vi "Device Pre Install Tasks.vi"(8 "Error In":errorcluster, 11 "Install LV Data":T1) -> (0 "Error Out":errorcluster, 3 "Install LV Data":T1={"SSH Session"=refnum, "Status Log"="", "Detailed Log"="", "Credentials"={"Hostname or IP"="192.168.7.2", "Username"="root", "Password"=""}, "Target Info"={"OS Version"="", "CPU"="", "Systemd Version"="", "Internet Access"=FALSE, "Device Type"="", "LV Installed Ver"="", "LV Available Ver"="", "LV Upgrade Available"=FALSE, "Hostname"="", "NIC Info"=[]}, "Reboot Required?"=FALSE})   [LabVIEW 2014, in "LMH-LINX.lvlib"]
uses:
  <vilib>/MakerHub/LINX/LMH-LINX.lvlib
  <vilib>/MakerHub/LINX/Private/Utilties/Target Management/Install LV Data.ctl
  C:/Program Files (x86)/National Instruments/LabVIEW 2014/vi.lib/MakerHub/LINX/Resources/Renci.SshNet.dll
  Resources/Renci.SshNet.dll
  <vilib>/MakerHub/LINX/Private/Utilties/Target Management/Target Info.ctl
  <vilib>/MakerHub/LINX/Private/Utilties/Target Management/NIC Info.ctl
  <vilib>/MakerHub/LINX/Private/Utilties/Target Management/NIC Mode.ctl
  <vilib>/MakerHub/LINX/Private/Utilties/Target Management/Status FGV States.ctl
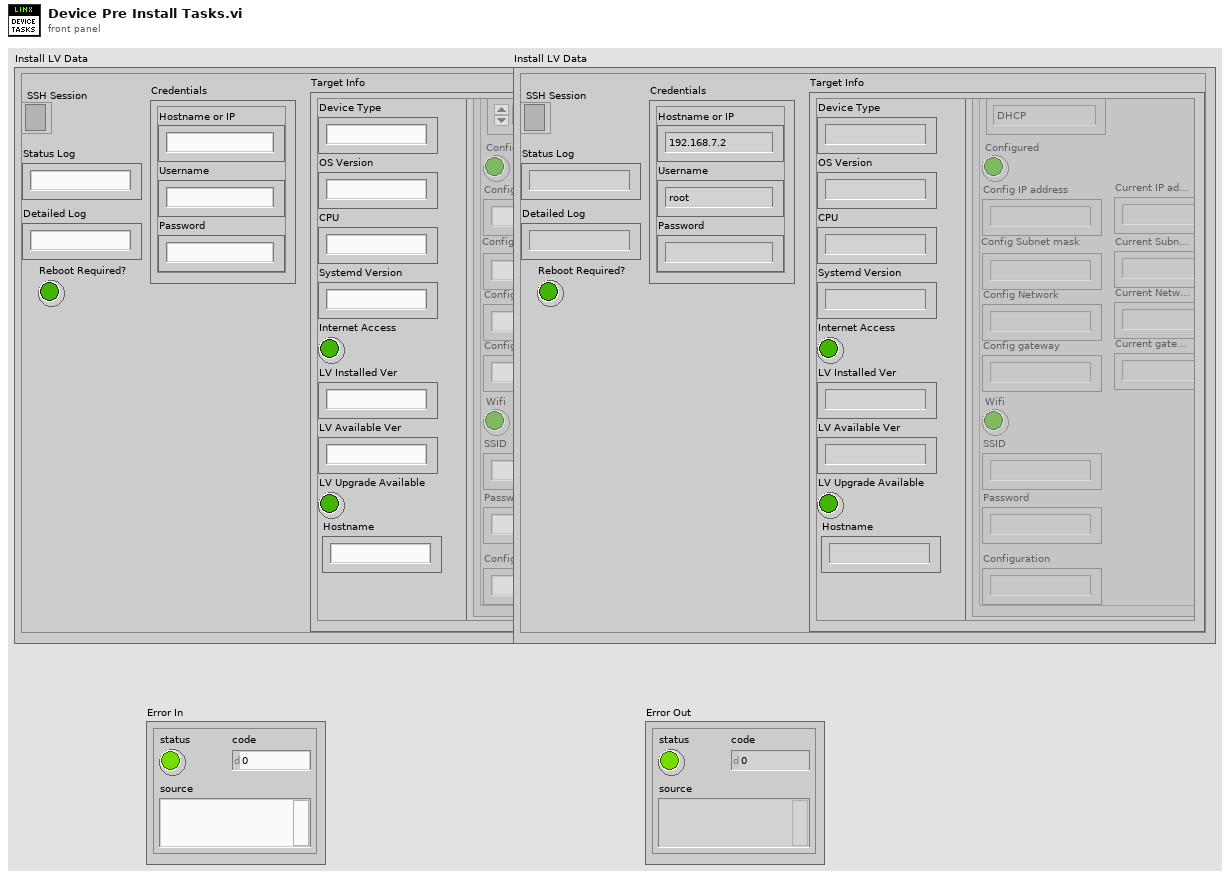
[diagram p1: front panel]
types:
  T1 = typedef "LMH-LINX.lvlib/Install LV Data.ctl" = cluster{"SSH Session":refnum<k24>, "Status Log":string, "Detailed Log":string, "Credentials":cluster{"Hostname or IP":string, "Username":string, "Password":string}, "Target Info":T2, "Reboot Required?":bool}
  T2 = typedef "LMH-LINX.lvlib/Target Info.ctl" = cluster{"OS Version":string, "CPU":string, "Systemd Version":string, "Internet Access":bool, "Device Type":string, "LV Installed Ver":string, "LV Available Ver":string, "LV Upgrade Available":bool, "Hostname":string, "NIC Info":T3[]}
  T3 = typedef "LMH-LINX.lvlib/NIC Info.ctl" = cluster{"Name":string, "NIC Mode":T4, "Configured":bool, "Config IP address":string, "Config Subnet mask":string, "Config Network":string, "Config gateway":string, "Wifi":bool, "SSID":string, "Password":string, "Configuration":string, "Current IP address":string, "Current Subnet mask":string, "Current gateway":string, "Current Network":string}
  T4 = typedef "LMH-LINX.lvlib/NIC Mode.ctl" = enum16{"DHCP", "Static", "Loopback"}
  T5 = typedef "LMH-LINX.lvlib/Status FGV States.ctl" = enum16{"Init", "Append", "Append History Only", "Set", "Get"}
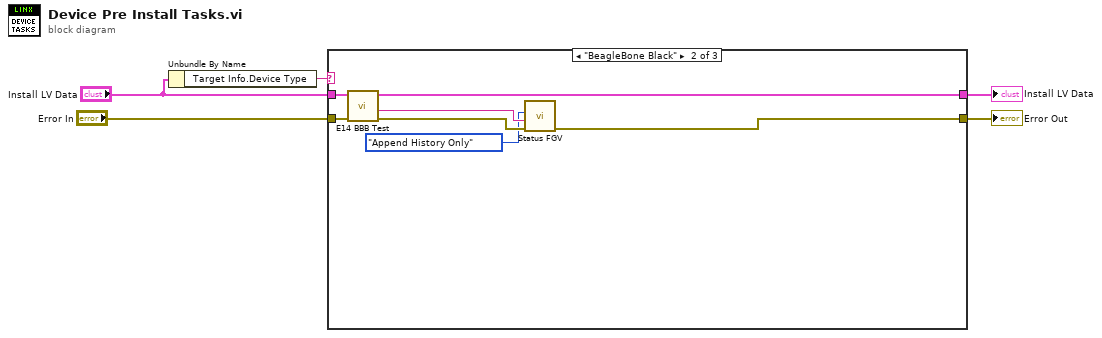
[diagram p0: block diagram]
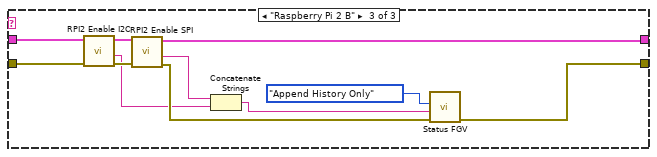
[diagram p3: hidden frame]
diagram:
  n1 = Unbundle By Name("Install LV Data") -> ("Target Info.Device Type"=w2:string)
  n2 = case shown="\"BeagleBone Black\"" w2 {
    tunnel: "Error In" -> [w7 w14 w23]
    tunnel: "Install LV Data" -> [w6 w13 w24]
    tunnel: [w7 w11 w25] -> w3
    tunnel: [w6 w8 w22] -> w1
    frame "False", Default {
    }
    frame "BeagleBone Black" {
      n3 = call <vilib>:"E14 BBB Test.vi"("Error In"=w14, "Install LV Data"=w13) -> ("Error Out"=w12:errorcluster, "Status"=w10:string, "Install LV Data"=w8:T1)  [unwired: 7 in]
      n4 = call <vilib>:"Status FGV.vi"("Error In"=w12, "Status"=w10, "Status FGV State"=Status_FGV_States."Append History Only") -> ("Error Out"=w11:errorcluster)  [unwired: 6 in, 2 out]
    }
    frame "Raspberry Pi 2 B" {
      n5 = call <vilib>:"RPI2 Enable I2C.vi"("Error In"=w23, "Install LV Data"=w24) -> ("Error Out"=w20:errorcluster, "Log"=w16:string, "Install LV Data"=w19:T1)  [unwired: 7 in]
      n6 = call <vilib>:"RPI2 Enable SPI.vi"("Error In"=w20, "Install LV Data"=w19) -> ("Error Out"=w18:errorcluster, "Log"=w17:string, "Install LV Data"=w22:T1)  [unwired: 7 in]
      n7 = Concatenate Strings(w17, w16) -> (w15:string)
      n8 = call <vilib>:"Status FGV.vi"("Error In"=w18, "Status"=w15, "Status FGV State"=Status_FGV_States."Append History Only") -> ("Error Out"=w25:errorcluster)  [unwired: 6 in, 2 out]
    }
  }
  "Error Out" <- w3
  "Install LV Data" <- w1
